vi "Determine Peek Stack Display.vi"(8 "error in":errorcluster, 11 "Module Data":T1) -> (0 "error out":errorcluster, 1 "Unique VI Names for Display":string[](array[string]), 2 "Tags":string[](array[string]), 3 "Module Data":T1)   [LabVIEW 2020, in "Peek Window.lvlib"]
uses:
  Peek Window.lvlib
  MHL Data Cluster.ctl
  Open Diagram Argument--cluster.ctl
  VI Types Enum.ctl
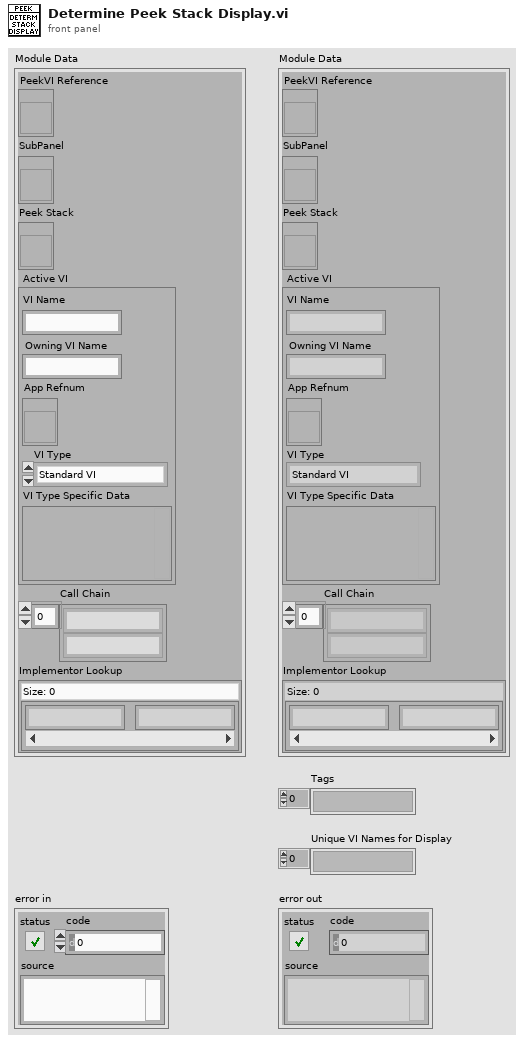
[diagram p1: front panel]
types:
  T1 = typedef "Peek Window.lvlib/MHL Data Cluster.ctl" = cluster{"PeekVI Reference":refnum<vi>, "SubPanel":refnum<vi>, "Peek Stack":refnum<vi>, "Active VI":T2, "Call Chain":string[], "Implementor Lookup":map{string, string}}
  T2 = typedef "Peek Window.lvlib/Open Diagram Argument--cluster.ctl" = cluster{"VI Name":string, "Owning VI Name":string, "App Refnum":refnum<vi>, "VI Type":T3, "VI Type Specific Data":variant}
  T3 = typedef "Peek Window.lvlib/VI Types Enum.ctl" = enum16{"Standard VI", "Dynamic Dispatch VI", "Malleable VI", "Express VI", "Polymorphic VI", "Missing VI"}
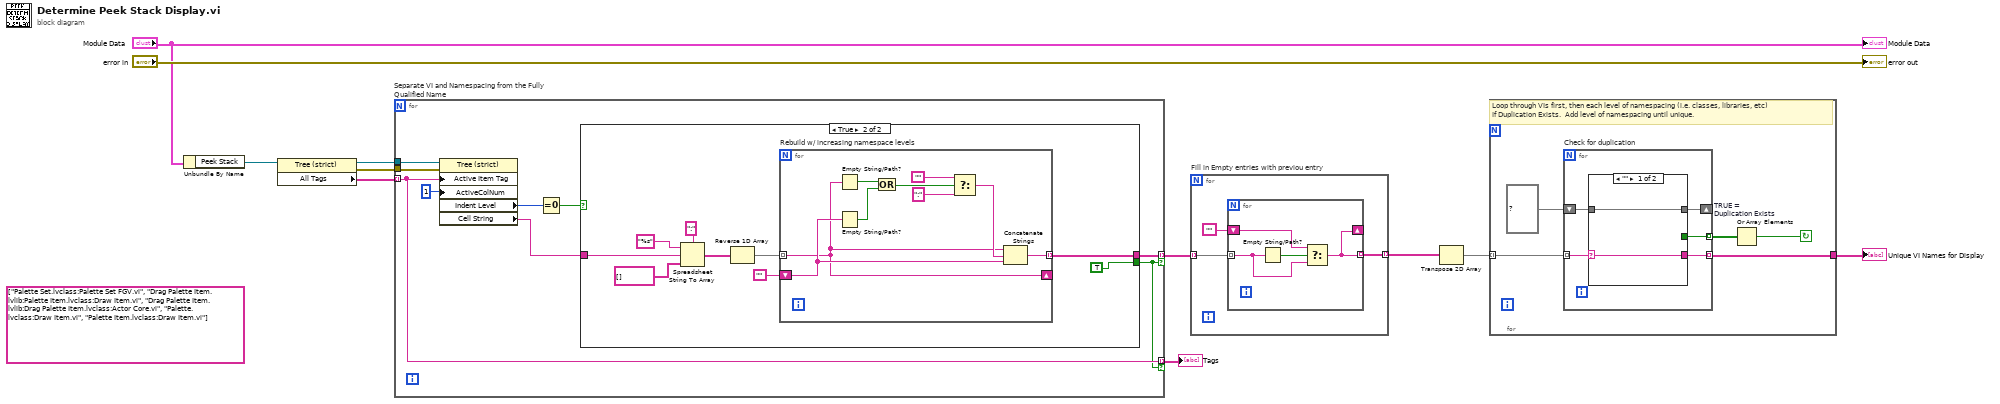
[diagram p0: block diagram]
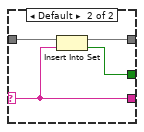
[diagram p3: hidden frame]
diagram:
  (unwired) string[] ["Palette Set.lvclass:Palette Set FGV.vi", "Drag Palette Item.lvlib:Palette Item.lvclass:Draw Item.vi", "Drag Palette Item.lvlib:Drag Palette Item.lvclass:Actor Core.vi", "Palette.lvclass:Draw Item.vi", "Palette Item.lvclass:Draw Item.vi"]
  n1 = Unbundle By Name("Module Data") -> ("Peek Stack"=w6:refnum<vi>)
  n2 = property class="Tree (strict)"(reference=w6) -> (reference out=w4:refnum<vi>, error out=w3:errorcluster, "All Tags"=w5:string[])  [unwired: 1 in]
  n3 = for "Separate VI and Namespacing from the Fully Qualified Name" {
    tunnel: [w20] -> w9 mode=indexing if=w12
    tunnel: w5 -> [w13] mode=indexing
    tunnel: w4 -> [w19]
    tunnel: w3 -> [w18]
    tunnel: [w13] -> w1 mode=indexing if=w12
    n4 = property class="Tree (strict)"(reference=w19, error in=w18, "Active Item Tag"=w13, "ActiveColNum"=1) -> ("Indent Level"=w15:i32, "Cell String"=w16:string)  [unwired: 2 out]
    n5 = Equal To 0?(x=w15) -> (x = 0?=w14:bool)
    n6 = case shown="True" w14 {
      selector: w14 -> [w21 _]
      tunnel: [_ w24] -> w20
      tunnel: w16 -> [_ w23]
      tunnel: [w21 TRUE] -> w12
      frame False {
      }
      frame True {
        n7 = Spreadsheet String To Array(delimiter (Tab)=":", format string="%s", spreadsheet string=w23, array type (2D Dbl)=string[] []) -> (array=w27:string[])
        n8 = Reverse 1D Array(array=w27) -> (reversed array=w26:string[])
        n9 = for "Rebuild w/ increasing namespace levels" {
          tunnel: w26 -> [w34] mode=indexing
          shift-right: [w34] -> _
          shift-left: "" -> [w38]
          tunnel: [w39] -> w24 mode=indexing
          n10 = Empty String/Path?(string/path=w34) -> (empty?=w33:bool)
          n11 = Empty String/Path?(string/path=w38) -> (empty?=w32:bool)
          n12 = Or(x=w33, y=w32) -> (x .or. y?=w31:bool)
          n13 = Select(t="", s=w31, f=":") -> (s? t:f=w35:string)
          n14 = Concatenate Strings(w34, w35, w38) -> (w39:string)
        }
      }
    }
  }
  "Tags" <- w1
  n15 = for "Fill in Empty entries with previou entry" {
    tunnel: w9 -> [w42] mode=indexing
    tunnel: [w41] -> w8 mode=indexing
    n16 = for {
      tunnel: w42 -> [w45] mode=indexing
      tunnel: [w44] -> w41 mode=indexing
      shift-right: [w44] -> _
      shift-left: "" -> [w43]
      n17 = Empty String/Path?(string/path=w45) -> (empty?=w46:bool)
      n18 = Select(t=w43, s=w46, f=w45) -> (s? t:f=w44:string)
    }
  }
  n19 = Transpose 2D Array(2D array=w8) -> (transposed array=w11:string[][])
  n20 = for {
    tunnel: w11 -> [w51] mode=indexing
    tunnel: [w47] -> w10
    stop <- w48 continue-if-true
    # "Loop through VIs first, then each level of namespacing (i.e. classes, libraries, etc)\nIf Duplication Exists.  Add level of namespacing until unique."
    n21 = for "Check for duplication" {
      tunnel: w51 -> [w55] mode=indexing
      shift-right: [w53] -> _
      shift-left: set{string} {} ("set in") -> [w56]
      tunnel: [w54] -> w49 mode=indexing
      tunnel: [w52] -> w47 mode=indexing
      n22 = case shown="\"\"" w55 {
        selector: w55 -> [w57 w59]
        tunnel: w56 -> [w58 w61]
        tunnel: [_ w62] -> w54
        tunnel: [w58 w60] -> w53
        tunnel: [w57 w59] -> w52
        frame "" {
        }
        frame Default {
          n23 = Insert Into Set(10:w59, 11:w61) -> (2:w62:bool, 3:w60:set{string})
        }
      }
    }
    n24 = Or Array Elements "TRUE =\nDuplication Exists"(Boolean array=w49) -> (logical OR=w48:bool)
  }
  "Unique VI Names for Display" <- w10
  "Module Data" <- "Module Data"
  "error out" <- "error in"
